vi "Merge Similar.vi"(1 "AA Instructions":i32[][](array[numeric])) -> (0 "Merged Instructions":i32[][](array[numeric]))   [LabVIEW 2015]
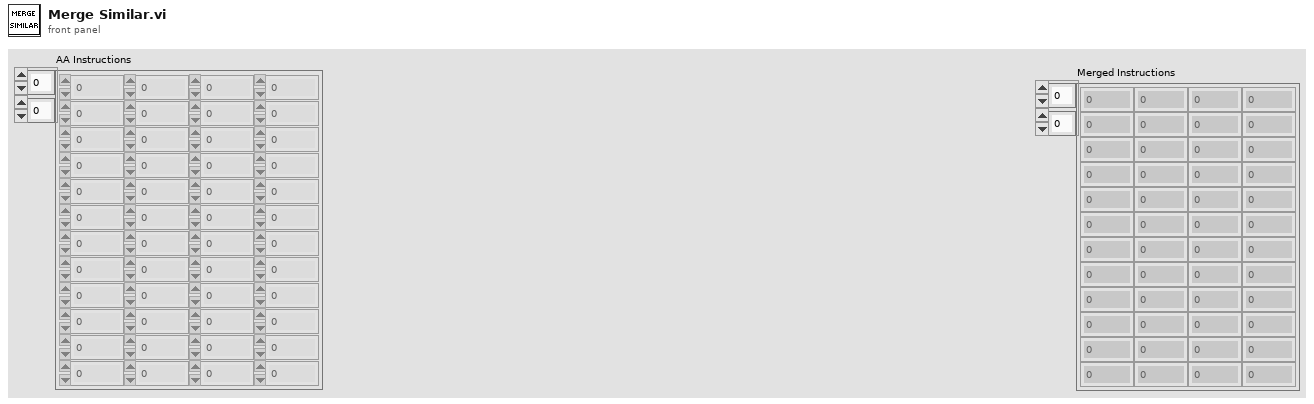
[diagram p1: front panel]
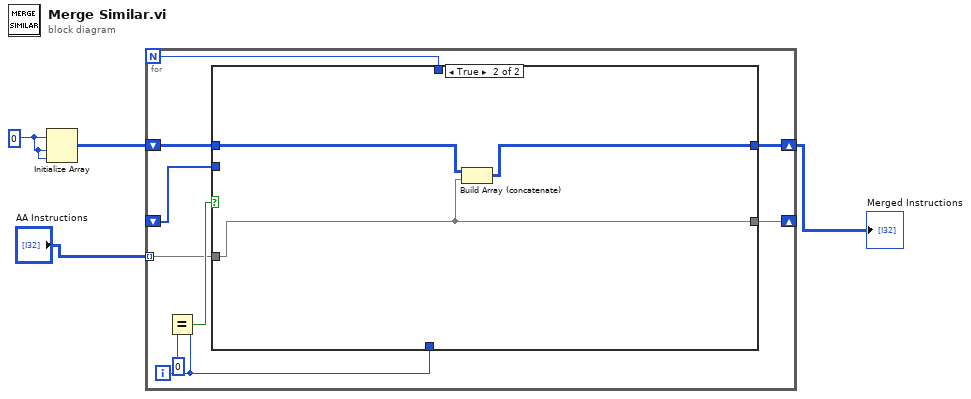
[diagram p0: block diagram]
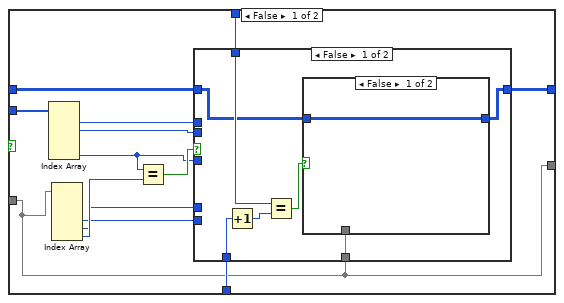
[diagram p2: hidden frame]
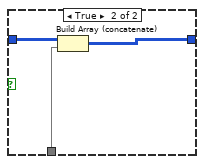
[diagram p3: hidden frame]
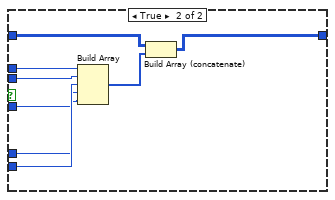
[diagram p4: hidden frame]
diagram:
  w3 = 0
  n1 = Initialize Array(w3, w3, w3) -> (w2:i32[][])
  n2 = for {
    N -> [w6]
    shift-right: [w10] -> _
    shift-left: _ -> [w9]
    tunnel: "AA Instructions" -> [w11] mode=indexing
    shift-right: [w7] -> w1
    shift-left: w2 -> [w8]
    i -> [w5]
    n3 = Equal?(x=w5, y=0) -> (x = y?=w12:bool)
    n4 = case shown="True" w12 {
      tunnel: w11 -> [w14 w46]
      tunnel: [w14 w46] -> w10
      tunnel: w9 -> [w26 _]
      tunnel: w8 -> [w23 w48]
      tunnel: [w22 w47] -> w7
      tunnel: w6 -> [w16 _]
      tunnel: w5 -> [w15 _]
      frame False {
        n5 = Index Array(array=w26) -> (element #1=w21:i32, element #2=w20:i32, element #5=w17:i32)  [unwired: 5 in, 2 out]
        n6 = Index Array(array=w14) -> (element #3=w19:i32, element #4=w18:i32, element #5=w25:i32)  [unwired: 5 in, 2 out]
        n7 = Equal?(x=w17, y=w25) -> (x = y?=w24:bool)
        n8 = case shown="False" w24 {
          tunnel: w23 -> [w29 w45]
          tunnel: [w28 w44] -> w22
          tunnel: w21 -> [_ w43]
          tunnel: w20 -> [_ w42]
          tunnel: w19 -> [_ w41]
          tunnel: w18 -> [_ w40]
          tunnel: w17 -> [_ w39]
          tunnel: w16 -> [w33 _]
          tunnel: w15 -> [w31 _]
          tunnel: w14 -> [w27 _]
          frame False {
            n9 = Increment(x=w31) -> (x+1=w32:i32)
            n10 = Equal?(x=w33, y=w32) -> (x = y?=w30:bool)
            n11 = case shown="False" w30 {
              tunnel: w29 -> [w34 w37]
              tunnel: [w34 w36] -> w28
              tunnel: w27 -> [_ w35]
              frame False {
              }
              frame True {
                n12 = Build Array (concatenate)(w37, w35) -> (w36:i32[][])
              }
            }
          }
          frame True {
            n13 = Build Array(w43, w42, w41, w40, w39) -> (w38:i32[])
            n14 = Build Array (concatenate)(w45, w38) -> (w44:i32[][])
          }
        }
      }
      frame True {
        n15 = Build Array (concatenate)(w48, w46) -> (w47:i32[][])
      }
    }
  }
  "Merged Instructions" <- w1
